vi "TDT-Read DI Buffers.vi"(0 "RPcox":refnum<k7>, 5 "Next Buffer":i32, 7 "Pts Per Read":i32, 9 "DI Channels":i32[](array[numeric])=[1, 2], 11 "error in (no error)":errorcluster, 12 "#inputs":i32) -> (8 "Input array":dbl[][](array[numeric]), 15 "error out":errorcluster)   [LabVIEW 2020]
panel:
  out "GetTagVal":sgl
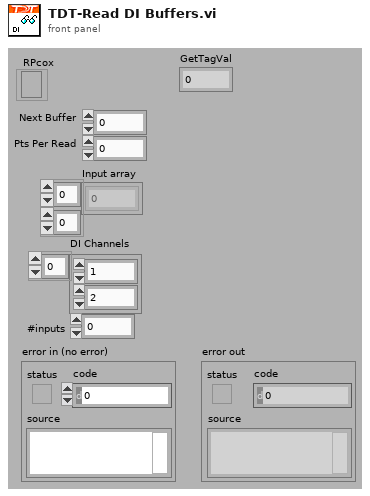
[diagram p1: front panel]
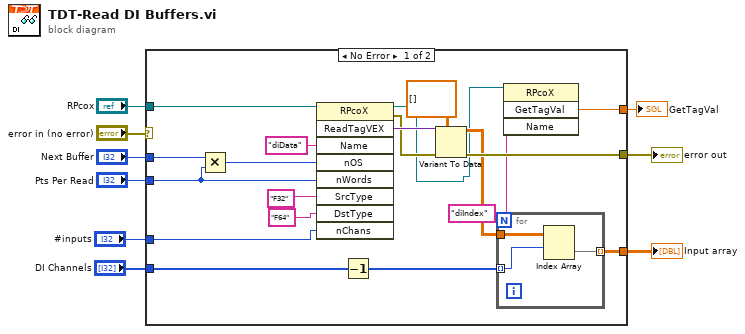
[diagram p0: block diagram]
diagram:
  n1 = case shown="No Error" "error in (no error)" {
    selector: "error in (no error)" -> [_ w32]
    tunnel: "Next Buffer" -> [w28 _]
    tunnel: "RPcox" -> [w27 _]
    tunnel: [w26 w32] -> w6
    tunnel: "Pts Per Read" -> [w20 _]
    tunnel: [w19 _] -> w4
    tunnel: "DI Channels" -> [w18 _]
    tunnel: "#inputs" -> [w13 _]
    tunnel: [w10 _] -> w1
    frame No Error {
      n2 = Multiply(x=w28, y=w20) -> (x*y=w21:i32)
      n3 = invoke class="RPcoX" method="ReadTagVEX"(reference=w27, "Name"="diData", "nOS"=w21, "nWords"=w20, "SrcType"="F32" ("DstType"), "DstType"="F64", "nChans"=w13) -> (reference out=w11:refnum<k7>, error out=w23:errorcluster, "ReadTagVEX"=w25:variant)  [unwired: 2 in, 6 out]
      n4 = Decrement(x=w18) -> (x-1=w16:i32[])
      n5 = Variant To Data(error in=w23, type=dbl[][] [] ("Input array"), Variant=w25) -> (data=w17:dbl[][], error out=w26:errorcluster)
      n6 = for {
        tunnel: w17 -> [w31]
        tunnel: [w30] -> w19 mode=indexing
        tunnel: w16 -> [w29] mode=indexing
        n7 = Index Array(array=w31, index (row)=w29) -> (element=w30:dbl[])  [unwired: 1 in]
      }
      n8 = invoke class="RPcoX" method="GetTagVal"(reference=w11, "Name"="diIndex" ("format string")) -> ("GetTagVal"=w10:sgl)  [unwired: 2 in, 3 out]
    }
    frame Error {
    }
  }
  "Input array" <- w4
  "error out" <- w6
  "GetTagVal" <- w1
